vi "Compute Flywheel Instantaneous Values.vi"(9 "Initial RPM":dbl, 11 "Motor Type":T3=enum."Neo") -> ()   [LabVIEW 2019]
uses:
  Motor Type.ctl
  Modeling/Battery Coefficients.ctl
  <vilib>/addons/control/pid/pid.llb/PID (DBL).vi
  <vilib>/addons/control/pid/NI_PID_pid.lvlib
panel:
  in  "Breaker":dbl[unit]=30.0
  in  "Battery Characterization":T1={"Battery Voltage"=12.9, "Internal Resistance"=0.015, "Battery Capacity"=64800.0, "Battery Temp"=75.0, "Battery Weight"=5.4431084400000005, "State of Charge %"=12.0} {"State of Charge %" format="%#_13g"; "Battery Weight" format="%#_13g"; "Battery Temp" format="%#_13g"; "Battery Capacity" format="%#_13g"; "Internal Resistance" format="%#_13g"; "Battery Voltage" format="%#_13g"}
  in  "stop":bool
  in  "Gear Ratio (out/in)":dbl=0.2
  in  "Flywheel Coefficients":T2={"Mass"=0.45359237, "Radius"=0.0508, "Coefficient (https://en.wikipedia.org/wiki/List_of_moments_of_inertia)"=0.7, "Name"="shooter wheel"}
  in  "Timestep":dbl[unit]=0.001 format="%#_3p"
  in  "Control":enum32{"Manual", "! !", "PID"}(tab)
  in  "Vbus %":dbl(slide)=27.27272727272728 scale=-100.0..100.0
  in  "When below":dbl[unit]=9.0
  in  "When Above":dbl[unit]
  in  "PID gains":T4={"proportional gain (Kc)"=1.9999999999999987, "integral time (Ti, min)"=0.0, "derivative time (Td, min)"=0.0} {"derivative time (Td, min)" format="%.3f"; "integral time (Ti, min)" format="%.3f"; "proportional gain (Kc)" format="%.3f"}
  in  "Setpoint RPM":dbl(slide)=4000.0 scale=-5676.0..5676.0
  out "Chart":T5(graph)
  # "Motor Information"
  # "Flywheel Information"
  # "Battery Information"
  # "Simulation Information"
  # "Simulation"
  # "RPM\n\nMotor V\n\nCurrent\n\nBatt V\n\nBreaker"
  # "Add breaker state"
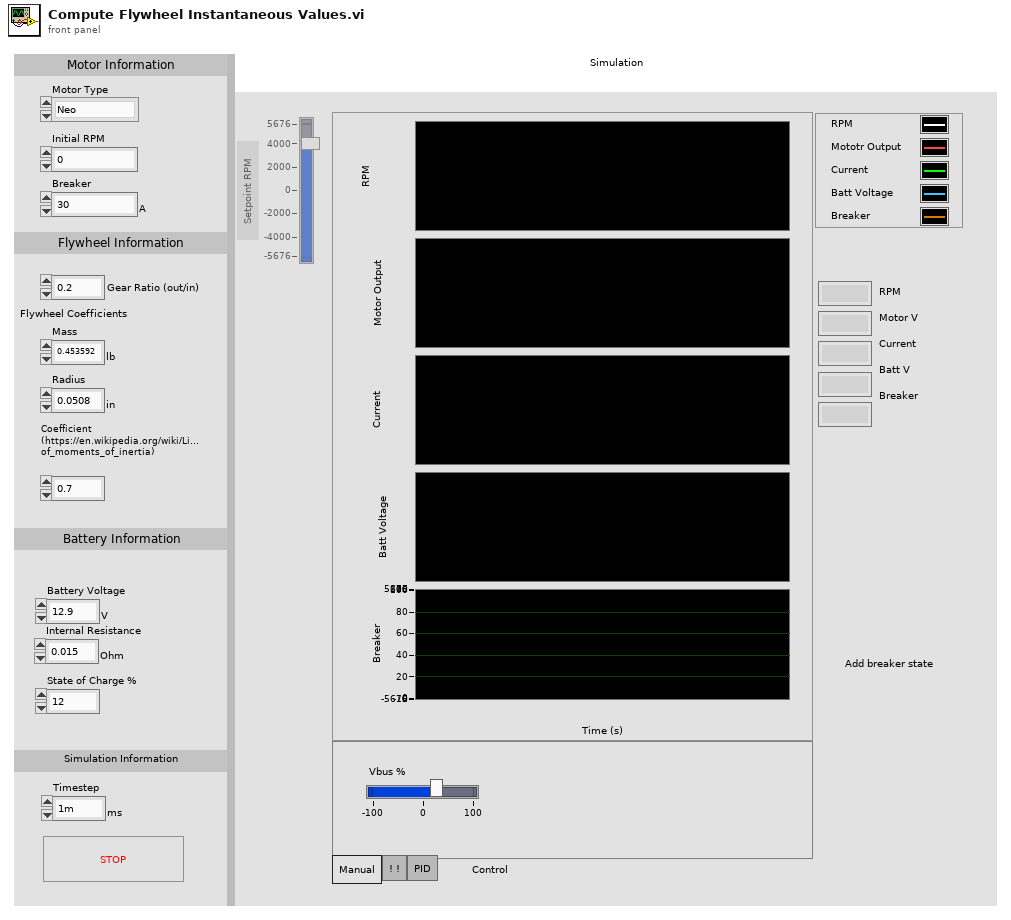
[diagram p1: front panel]
types:
  T1 = typedef "Battery Coefficients.ctl" = cluster{"Battery Voltage":dbl[unit], "Internal Resistance":dbl[unit], "Battery Capacity":dbl[unit], "Battery Temp":dbl[unit], "Battery Weight":dbl[unit], "State of Charge %":dbl}
  T2 = cluster{"Mass":dbl[unit], "Radius":dbl[unit], "Coefficient (https://en.wikipedia.org/wiki/List_of_moments_of_inertia)":dbl, "Name":string}
  T3 = typedef "Motor Type.ctl" = enum16{"Custom", "775 pro", "CIM", "miniCIM", "Neo", "Neo 550", "Falcon 500"}
  T4 = cluster{"proportional gain (Kc)":dbl, "integral time (Ti, min)":dbl, "derivative time (Td, min)":dbl}
  T5 = cluster{"Initial RPM":dbl, "When Above":dbl[unit], dbl[unit], "Battery Voltage":dbl[unit], dbl}
  T6 = cluster{"Initial RPM":dbl, "When Above":dbl[unit], dbl[unit], "Battery Voltage":dbl[unit], dbl}[]
  T7 = typedef "Motor Physical Values.ctl" = cluster{"Ratio (out/in)":dbl, "Moment of Inertia (kg m^2)":dbl[unit]}
  T8 = typedef "Motor Operating Values.ctl" = cluster{"Kv":dbl[unit], "R":dbl[unit], "Kt":dbl[unit], "Breaker Size":dbl[unit]}
  T9 = enum8{"Enabled", "Disabled", "Disabled and Grayed Out"}
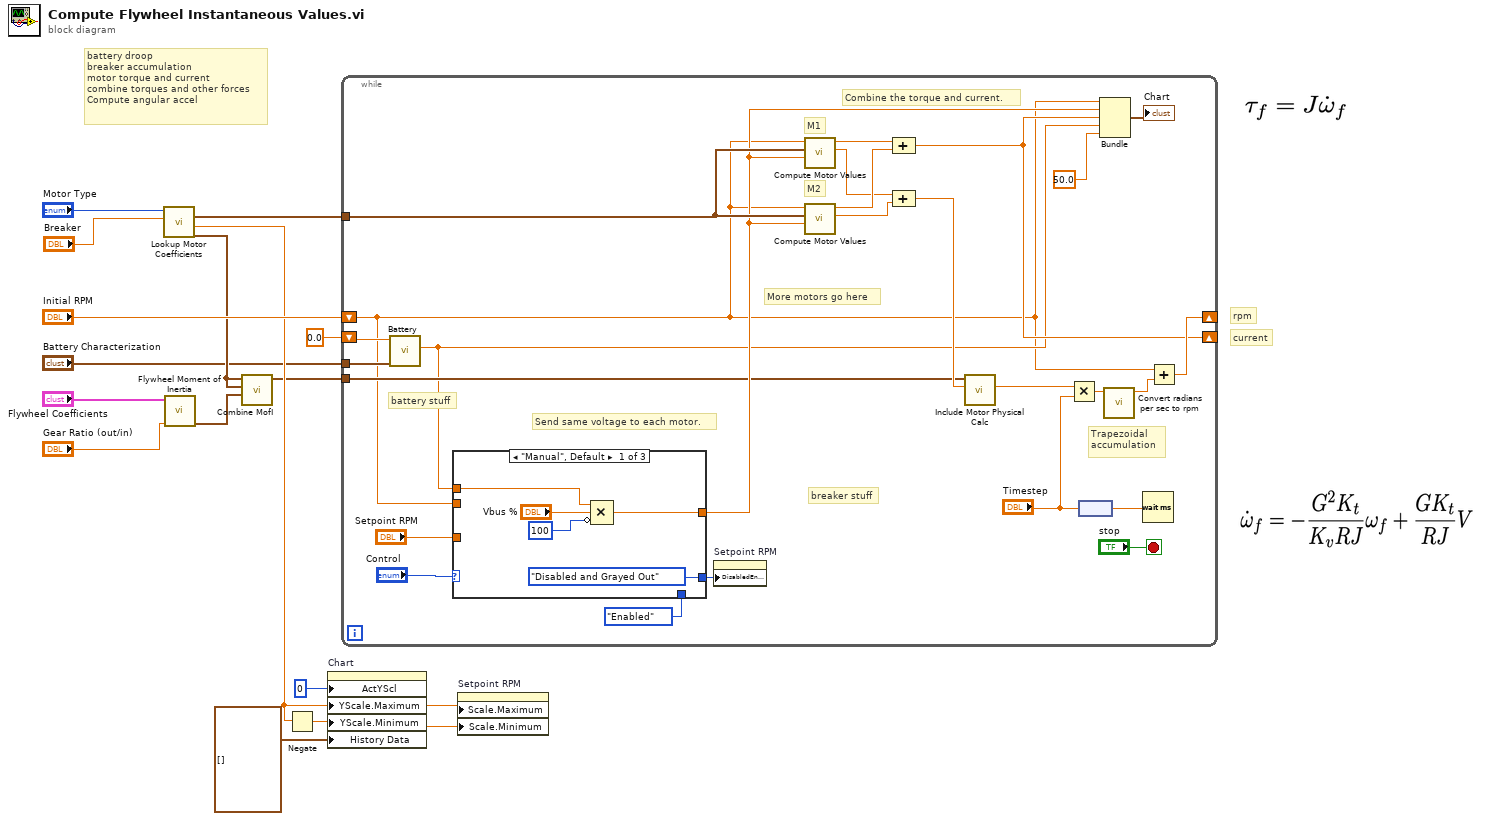
[diagram p0: block diagram]
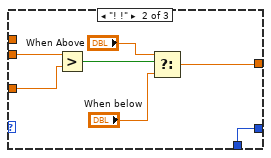
[diagram p2: hidden frame]
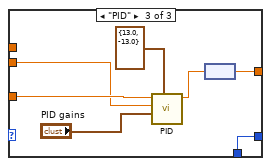
[diagram p3: hidden frame]
diagram:
  # "current"
  # "rpm"
  # "battery droop\nbreaker accumulation\nmotor torque and current\ncombine torques and other forces\nCompute angular accel"
  n1 = call "Lookup Motor Coefficients.vi"("Breaker Size"="Breaker", "Motor Type"="Motor Type") -> ("Physical Values"=w6:T7, "Free Speed"=w9:dbl, "Motor Model Values"=w14:T8)  [unwired: 6 in, 1 out]
  n2 = call "Flywheel Moment of Inertia.vi"("Gear Ratio (out/in)"="Gear Ratio (out/in)", "Flywheel Coefficients"="Flywheel Coefficients") -> ("Physical Values"=w5:T7)  [unwired: 9 in]
  n3 = call "Combine MofI.vi"("Rotational Mass 3"=w5, "Rotational Mass 2"=w6, "Rotational Mass 1"=w6) -> ("Combined"=w4:T7)  [unwired: 8 in]
  n4 = Negate(x=w9) -> (-x=w8:dbl)
  n5 = property on="Chart" class="WFChart (strict)"("ActYScl"=0 ("Active Y Scale"), "YScale.Maximum"=w9, "YScale.Minimum"=w8, "History Data"=T6 []) -> ()  [unwired: 2 in, 2 out]
  n6 = while {
    tunnel: w14 -> [w24]
    shift-right: [w41] -> _
    shift-left: "Initial RPM" -> [w17]
    tunnel: w4 -> [w20]
    shift-right: [w22] -> _
    shift-left: dbl[unit] 0.0 ("Current") -> [w29]
    tunnel: "Battery Characterization" -> [w18]
    stop <- "stop" stop-if-true
    # "Combine the torque and current."
    # "Trapezoidal\naccumulation"
    # "More motors go here"
    # "M2"
    # "M1"
    # "Send same voltage to each motor."
    # "breaker stuff"
    # "battery stuff"
    n7 = call "Battery.vi"("Battery Characterization"=w18, "Current"=w29) -> ("Battery Voltage"=w19:dbl[unit])  [unwired: 9 in]
    n8 = case shown="\"Manual\", Default" "Control" {
      tunnel: [w45 w50 w55] -> w23
      tunnel: w17 -> [_ w53 w58]
      tunnel: "Setpoint RPM" -> [_ w48 w59]
      tunnel: [T9."Disabled and Grayed Out" ("Disabled") w47 w54] -> w30
      tunnel: T9."Enabled" ("Disabled") -> [_ w47 w54]
      tunnel: w19 -> [w42 _ _]
      frame "Manual", Default {
        n9 = Compound Arithmetic op=MULTIPLY(w42, "Vbus %", invert 100) -> (w45:dbl[unit])
      }
      frame "! !" {
        n10 = Greater?(x=w53, y=w48) -> (0:w52:bool)
        n11 = Select(t="When Above", s=w52, f="When below") -> (s? t:f=w50:dbl[unit])
      }
      frame "PID" {
        n12 = call-poly <vilib>:"PID.vi"("output range"=cluster{"output high":dbl, "output low":dbl} {"output high"=13.0, "output low"=-13.0}, "PID gains"="PID gains", "process variable"=w58, "setpoint"=w59) -> ("output"=w56:dbl)  [unwired: 6 in, 1 out]
        n13 = node(w56) -> (w55:dbl[unit])
      }
    }
    n14 = property on="Setpoint RPM" class="Slide (strict)"("DisabledEnum"=w30) -> ()  [unwired: 2 in, 2 out]
    n15 = call "Compute Motor Values.vi"("Effective Motor Voltage"=w23, "Motor Model Values"=w24, "motor speed (rpm)"=w17) -> ("Motor Torque"=w26:dbl[unit], "Current"=w28:dbl[unit])  [unwired: 6 in, 1 out]
    n16 = call "Compute Motor Values.vi"("Effective Motor Voltage"=w23, "Motor Model Values"=w24, "motor speed (rpm)"=w17) -> ("Motor Torque"=w25:dbl[unit], "Current"=w27:dbl[unit])  [unwired: 6 in, 1 out]
    n17 = Compound Arithmetic op=ADD(w28, w27) -> (w22:dbl[unit])
    n18 = Compound Arithmetic op=ADD(w26, w25) -> (w21:dbl[unit])
    n19 = call "Include Motor Physical Calc.vi"("Motor Torque"=w21, "Physical Values"=w20) -> ("Angular Accel"=w35:dbl[unit])  [unwired: 8 in, 1 out]
    n20 = Multiply(x=w35, y="Timestep") -> (x*y=w39:dbl[unit])
    n21 = node("Timestep") -> (w36:dbl)
    n22 = Bundle("Initial RPM"=w17, "When Above"=w23, w22, "Battery Voltage"=w19, 50.0) -> (→"Chart":T5)  [unwired: 1 in]
    n23 = call "Convert radians per sec to rpm.vi"("speed in"=w39) -> ("speed out (rpm)"=w40:dbl)  [unwired: 10 in]
    n24 = Wait (ms)(milliseconds to wait=w36) -> ()  [unwired: 1 out]
    n25 = Add(x=w17, y=w40) -> (x+y=w41:dbl)
  }
  n26 = property on="Setpoint RPM" class="Slide (strict)"("Scale.Maximum"=w9, "Scale.Minimum"=w8) -> ()  [unwired: 2 in, 2 out]
